vi "Variable Launch Angle and Distance Trajectory.vi"() -> ()   [LabVIEW 2016]
panel:
  out "Horizontal Distance":dbl
  out "Time":dbl
  out "Target Speed":dbl
  out "Launch Angle":dbl
  out "Launch Y Velocity":dbl
  out "Launch X Velocity":dbl
  in  "Impact Angle":dbl(knob) scale=-1.5707963267948966..1.5707963267948966
  in  "Launch Speed":dbl(slide) scale=0.0..20.0
  in  "Height":dbl(slide) scale=0.0..10.0
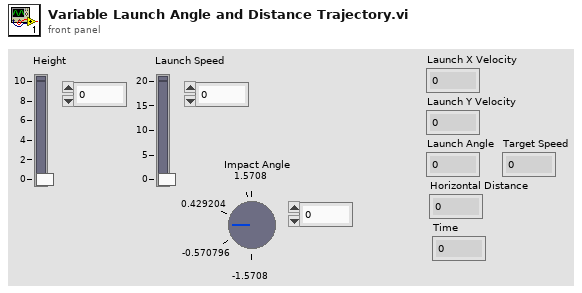
[diagram p1: front panel]
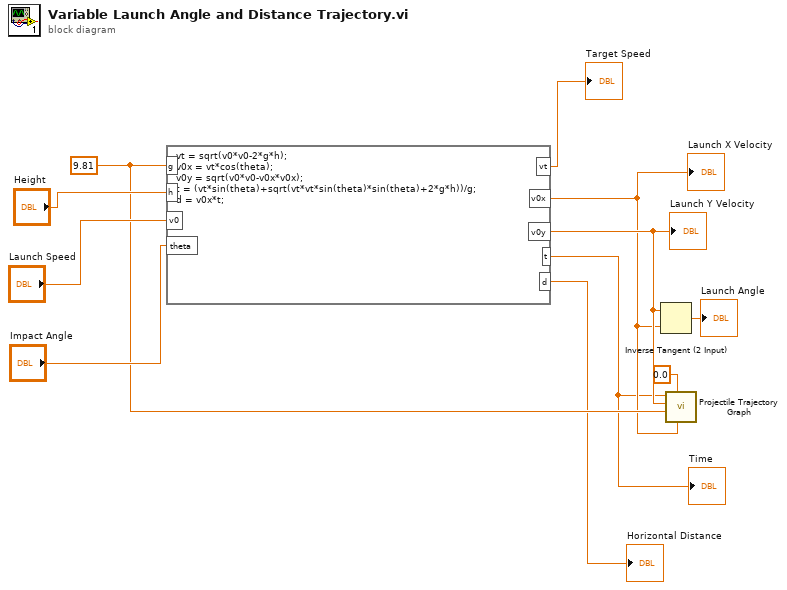
[diagram p0: block diagram]
diagram:
  w5 = 9.81 ("input variable")
  n1 = formula code="vt = sqrt(v0*v0-2*g*h);\nv0x = vt*cos(theta);\nv0y = sqrt(v0*v0-v0x*v0x);\nt = (vt*sin(theta)+sqrt(vt*vt*sin(theta)*sin(theta)+2*g*h))/g;\nd = v0x*t;"("g"=w5, "h"="Height", "v0"="Launch Speed", "theta"="Impact Angle") -> ("v0x"=w4:dbl, "v0y"=w6:dbl, "vt"=→"Target Speed":dbl, "t"=w3:dbl, "d"=→"Horizontal Distance":dbl)
  "Launch X Velocity" <- w4
  "Launch Y Velocity" <- w6
  "Time" <- w3
  n2 = Inverse Tangent (2 Input)(1:w4, 2:w6) -> (0:→"Launch Angle":dbl)
  n3 = call "Projectile Trajectory Graph.vi"("X Velocity"=w4, "Initial Height"=0.0, "Gravitational Acceleration"=w5, "Initial Y Velocity"=w6, "End Time"=w3) -> ()  [unwired: 6 in, 1 out]
